vi "Refnums.vi"() -> ()   [LabVIEW 2014]
panel:
  in  "Arm Control":string="californiagirls"
  in  "Conver B":string="Murder"
  in  "Conver T":string="redruM"
  in  "Motors":string="wonderham"
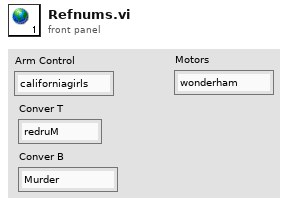
[diagram p1: front panel]
diagram:
